vi "test_cluster.vi"() -> ()   [LabVIEW 2019]
uses:
  test_cluster.ctl
panel:
  in  "Cluster":T1
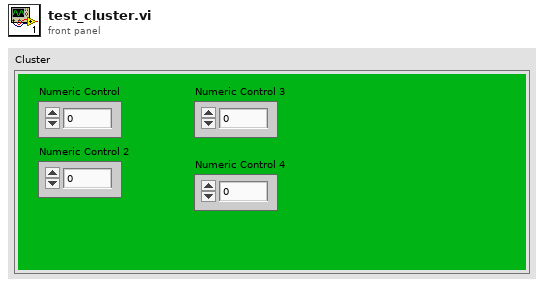
[diagram p1: front panel]
types:
  T1 = typedef "test_cluster.ctl" = cluster{"Numeric Control":dbl, "Numeric Control 2":dbl, "Numeric Control 3":dbl, "Numeric Control 4":dbl}
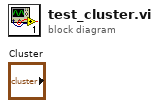
[diagram p0: block diagram]
diagram:
